vi "Configure Math Function (FFT).vi"(4 "Math Function Index (1: Math Function 1)":i32(ring)=1 items=["Math Function 1"=1, "Math Function 2"=2, "Math Function 3"=3, "Math Function 4"=4], 6 "FFT Vertical Units (0: Decibel)":i32(ring) items=["Decibel", "VRMS", "Degrees", "Radians"], 7 "Window Function (0: Rectangular)":i32(ring) items=["Rectangular", "Hanning", "Flat Top", "Blackman-Harris"], 8 "error in (no error)":errorcluster, 9 "Frequency Span (100000.0 Hz)":dbl=100000.0, 10 "Center Frequency (50000.0 Hz)":dbl=50000.0, 11 "VISA resource name":refnum<visa-resource-name>) -> (0 "error out":errorcluster, 3 "VISA resource name out":refnum<visa-resource-name>)   [LabVIEW 2015, in "Agilent 2000 3000 X-Series.lvlib"]
doc: "Configures the math function FFT."
uses:
  Agilent 2000 3000 X-Series.lvlib
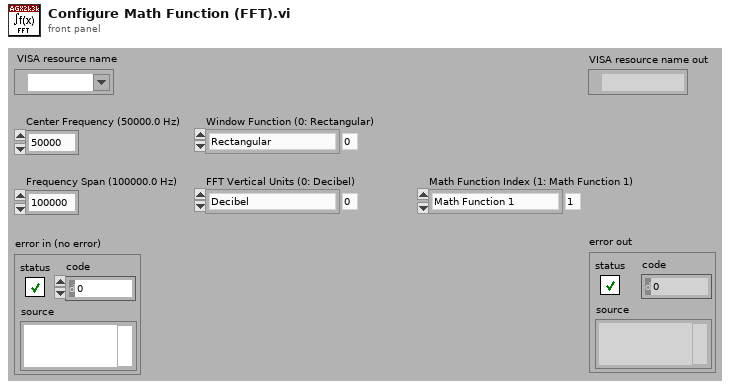
[diagram p1: front panel]
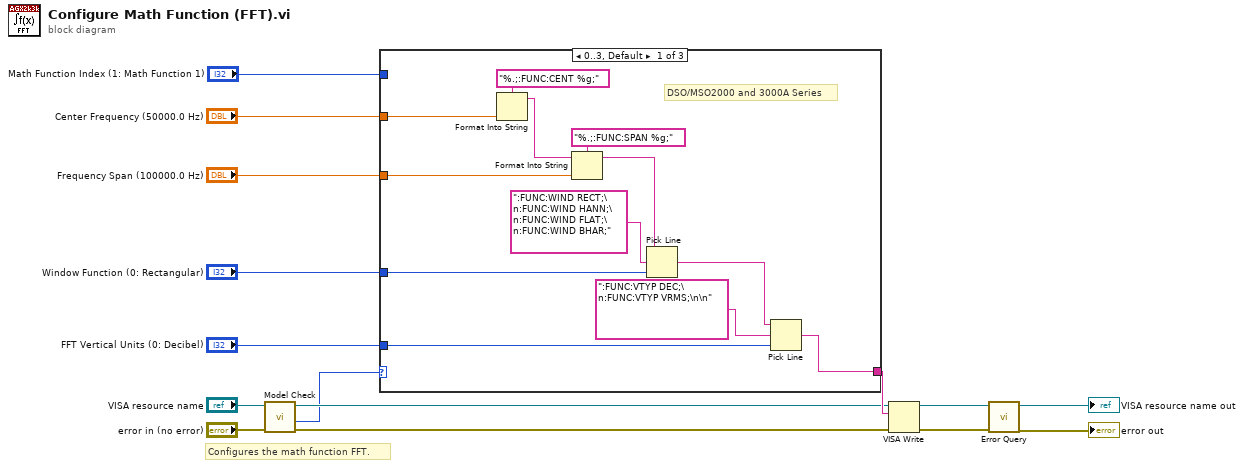
[diagram p0: block diagram]
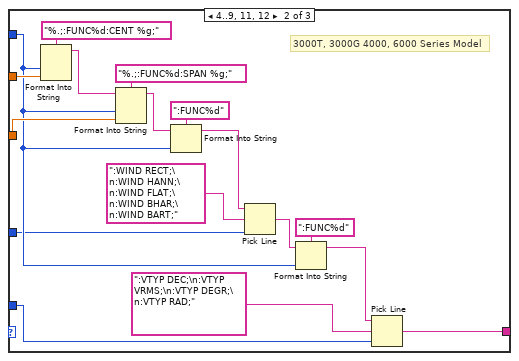
[diagram p2: hidden frame]
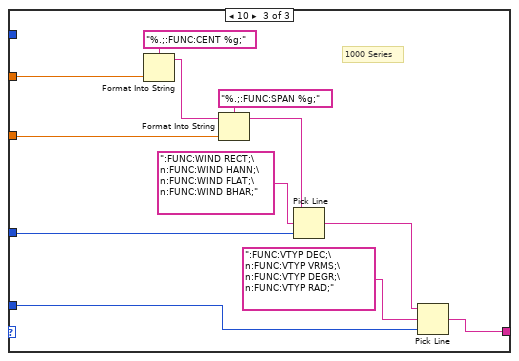
[diagram p3: hidden frame]
diagram:
  # "Configures the math function FFT."
  n1 = call "Model Check.vi"("error in (no error)"="error in (no error)", "VISA resource name"="VISA resource name") -> ("error out"=w3:errorcluster, "Model"=w1:i32, "VISA resource name out"=w4:refnum<visa-resource-name>)  [unwired: 7 out]
  n2 = case shown="0..3, Default" w1 {
    tunnel: "Center Frequency (50000.0 Hz)" -> [w26 w39 w47]
    tunnel: "Frequency Span (100000.0 Hz)" -> [w23 w38 w48]
    tunnel: "Window Function (0: Rectangular)" -> [w21 w31 w49]
    tunnel: "FFT Vertical Units (0: Decibel)" -> [w19 w30 w45]
    tunnel: [w16 w28 w46] -> w7
    tunnel: "Math Function Index (1: Math Function 1)" -> [_ w32 _]
    frame 0..3, Default {
      # "DSO/MSO2000 and 3000A Series"
      n3 = Format Into String(format string="%.;:FUNC:CENT %g;", w26) -> (resulting string=w25:string)  [unwired: 2 in, 1 out]
      n4 = Format Into String(format string="%.;:FUNC:SPAN %g;", initial string=w25, w23) -> (resulting string=w20:string)  [unwired: 1 in, 1 out]
      n5 = Pick Line(string ("")=w20, multi-line string=":FUNC:WIND RECT;\n:FUNC:WIND HANN;\n:FUNC:WIND FLAT;\n:FUNC:WIND BHAR;", line index=w21) -> (output string=w17:string)
      n6 = Pick Line(string ("")=w17, multi-line string=":FUNC:VTYP DEC;\n:FUNC:VTYP VRMS;\n\n", line index=w19) -> (output string=w16:string)
    }
    frame 4..9, 11, 12 {
      # "3000T, 3000G 4000, 6000 Series Model"
      n7 = Format Into String(format string="%.;:FUNC%d:CENT %g;", w32, w39) -> (resulting string=w43:string)  [unwired: 2 in, 1 out]
      n8 = Format Into String(format string="%.;:FUNC%d:SPAN %g;", initial string=w43, w32, w38) -> (resulting string=w36:string)  [unwired: 1 in, 1 out]
      n9 = Format Into String(format string=":FUNC%d", initial string=w36, w32) -> (resulting string=w35:string)  [unwired: 1 in, 1 out]
      n10 = Pick Line(string ("")=w35, multi-line string=":WIND RECT;\n:WIND HANN;\n:WIND FLAT;\n:WIND BHAR;\n:WIND BART;", line index=w31) -> (output string=w33:string)
      n11 = Format Into String(format string=":FUNC%d", initial string=w33, w32) -> (resulting string=w29:string)  [unwired: 1 in, 1 out]
      n12 = Pick Line(string ("")=w29, multi-line string=":VTYP DEC;\n:VTYP VRMS;\n:VTYP DEGR;\n:VTYP RAD;", line index=w30) -> (output string=w28:string)
    }
    frame 10 {
      # "1000 Series"
      n13 = Format Into String(format string="%.;:FUNC:CENT %g;", w47) -> (resulting string=w55:string)  [unwired: 2 in, 1 out]
      n14 = Format Into String(format string="%.;:FUNC:SPAN %g;", initial string=w55, w48) -> (resulting string=w52:string)  [unwired: 1 in, 1 out]
      n15 = Pick Line(string ("")=w52, multi-line string=":FUNC:WIND RECT;\n:FUNC:WIND HANN;\n:FUNC:WIND FLAT;\n:FUNC:WIND BHAR;", line index=w49) -> (output string=w50:string)
      n16 = Pick Line(string ("")=w50, multi-line string=":FUNC:VTYP DEC;\n:FUNC:VTYP VRMS;\n:FUNC:VTYP DEGR;\n:FUNC:VTYP RAD;", line index=w45) -> (output string=w46:string)
    }
  }
  n17 = VISA Write(VISA resource name=w4, write buffer=w7, error in (no error)=w3) -> (VISA resource name out=w12:refnum<visa-resource-name>, error out=w11:errorcluster)  [unwired: 1 out]
  n18 = call "Error Query.vi"("error in (no error)"=w11, "VISA resource name"=w12) -> ("error out"=→"error out":errorcluster, "VISA resource name out"=→"VISA resource name out":refnum<visa-resource-name>)  [unwired: 8 out]
